vi "HovaCal Stufen aufteilen.vi"(6 "Komponentenauswahl":cluster{"Komponente:":T1, "Konzentration":dbl} {"Konzentration" format="%#.6f"}, 7 "Punkte umkehren":bool, 8 "error in (no error)":errorcluster caption="Fehler (Eingang, kein Fehler)", 9 "Anzahl Stufen":T2 format="%#_5g", 11 "Gasteiler Stufen":T3=128 items=["10"=10, "11"=11, "16"=16, "32"=32, "64"=64, "128"=128, "256"=256, "500"=500, "1000"=1000]) -> (0 "error out":errorcluster caption="Fehler (Ausgang)", 1 "Stufen":dbl[](array[numeric]), 3 "Stufen":u16[](array[numeric]), 4 "Komponente:":T1)   [LabVIEW 2020, in "Linearisierung v2.lvlib" / "Gasteiler.lvlib" / "HovaCAL_Interface.lvlib"]
uses:
  HovaCAL_Interface.lvlib
  Gasteiler Stufen.ctl
  Visualisierungs Elemente/Zahlen-Eingabefeld.ctl
  Visualisierungs Elemente/Auswahlfeld.ctl
  Gasteiler.lvlib
  HovaCal/HovaCal.lvlib
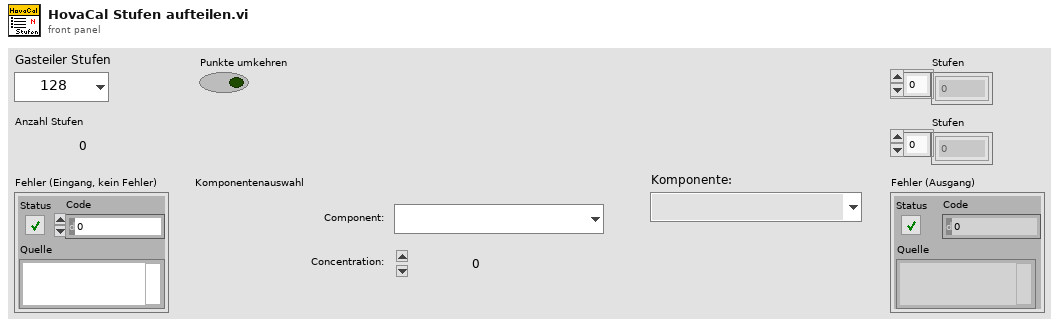
[diagram p1: front panel]
types:
  T1 = typedef "Auswahlfeld.ctl" = u16
  T2 = typedef "Zahlen-Eingabefeld.ctl" = sgl
  T3 = typedef "Linearisierung v2.lvlib/Gasteiler.lvlib/Gasteiler Stufen.ctl" = u16
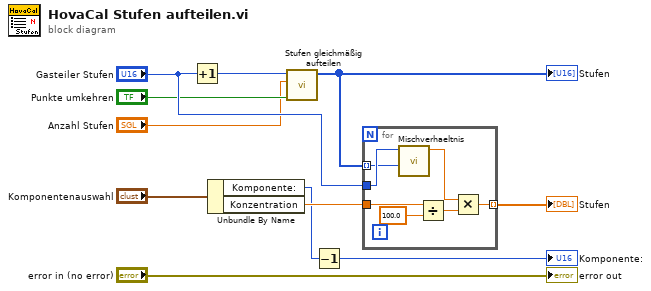
[diagram p0: block diagram]
diagram:
  n1 = Increment(x="Gasteiler Stufen") -> (x+1=w10:T3)
  n2 = Unbundle By Name("Komponentenauswahl") -> ("Komponente:"=w2:T1, "Konzentration"=w8:dbl)
  n3 = call "Stufen gleichmäßig aufteilen.vi"("Punkte umkehren"="Punkte umkehren", "Stufen"="Anzahl Stufen", "Anzahl"=w10) -> ("Stufen"=w11:u16[])  [unwired: 8 in]
  "Stufen" <- w11
  n4 = Decrement(x=w2) -> (x-1=→"Komponente:":T1)
  n5 = for {
    tunnel: w11 -> [w17] mode=indexing
    tunnel: "Gasteiler Stufen" -> [w18]
    tunnel: w8 -> [w16]
    tunnel: [w12] -> w9 mode=indexing
    n6 = call "Mischverhaeltnis.vi"("Konzentration"=w17, "Sollwert"=w18) -> ("%"=w13:dbl)  [unwired: 8 in, 1 out]
    n7 = Divide(x=w16, y=sgl 100.0) -> (x/y=w14:dbl)
    n8 = Multiply(x=w13, y=w14) -> (x*y=w12:dbl)
  }
  "Stufen" <- w9
  "error out" <- "error in (no error)"
